vi "Get Least Common Multiple (LCM)-array input.vi"(8 "Error In":errorcluster, 11 "Input integers":i32[](array[numeric])) -> (0 "Error Out":errorcluster, 3 "Least Common Multiple (LCM)":i32)   [LabVIEW 2021, in "Numeric Utilities.lvlib"]
uses:
  Numeric Utilities.lvlib
  Factors cluster.ctl
panel:
  out "Loop iteration":i32
  # "Development\ncontrols/indicators useful for development and testing, but which are not outputs of the VI"
  # "Input\nInputs to the VI"
  # "Output\nOutputs of the VI"
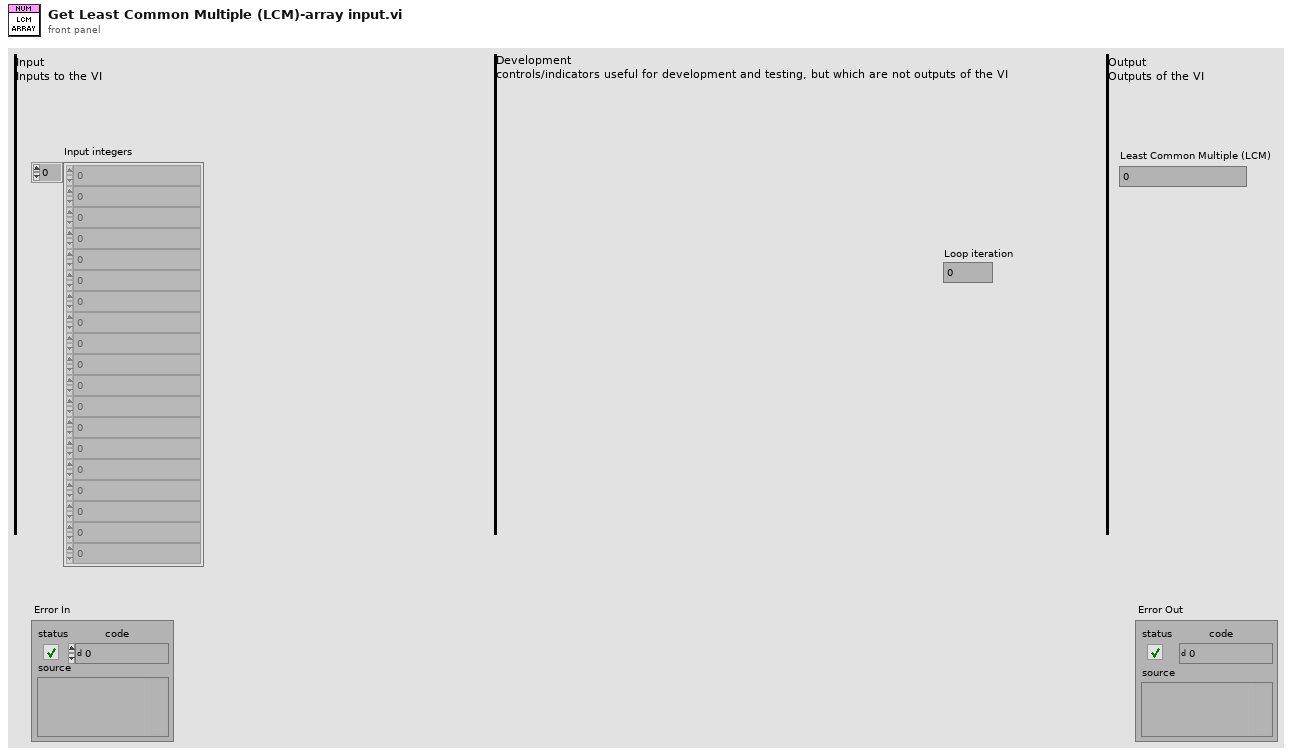
[diagram p1: front panel]
types:
  T1 = typedef "Numeric Utilities.lvlib/Factors cluster.ctl" = cluster{"Factor":i32, "Power":i32}
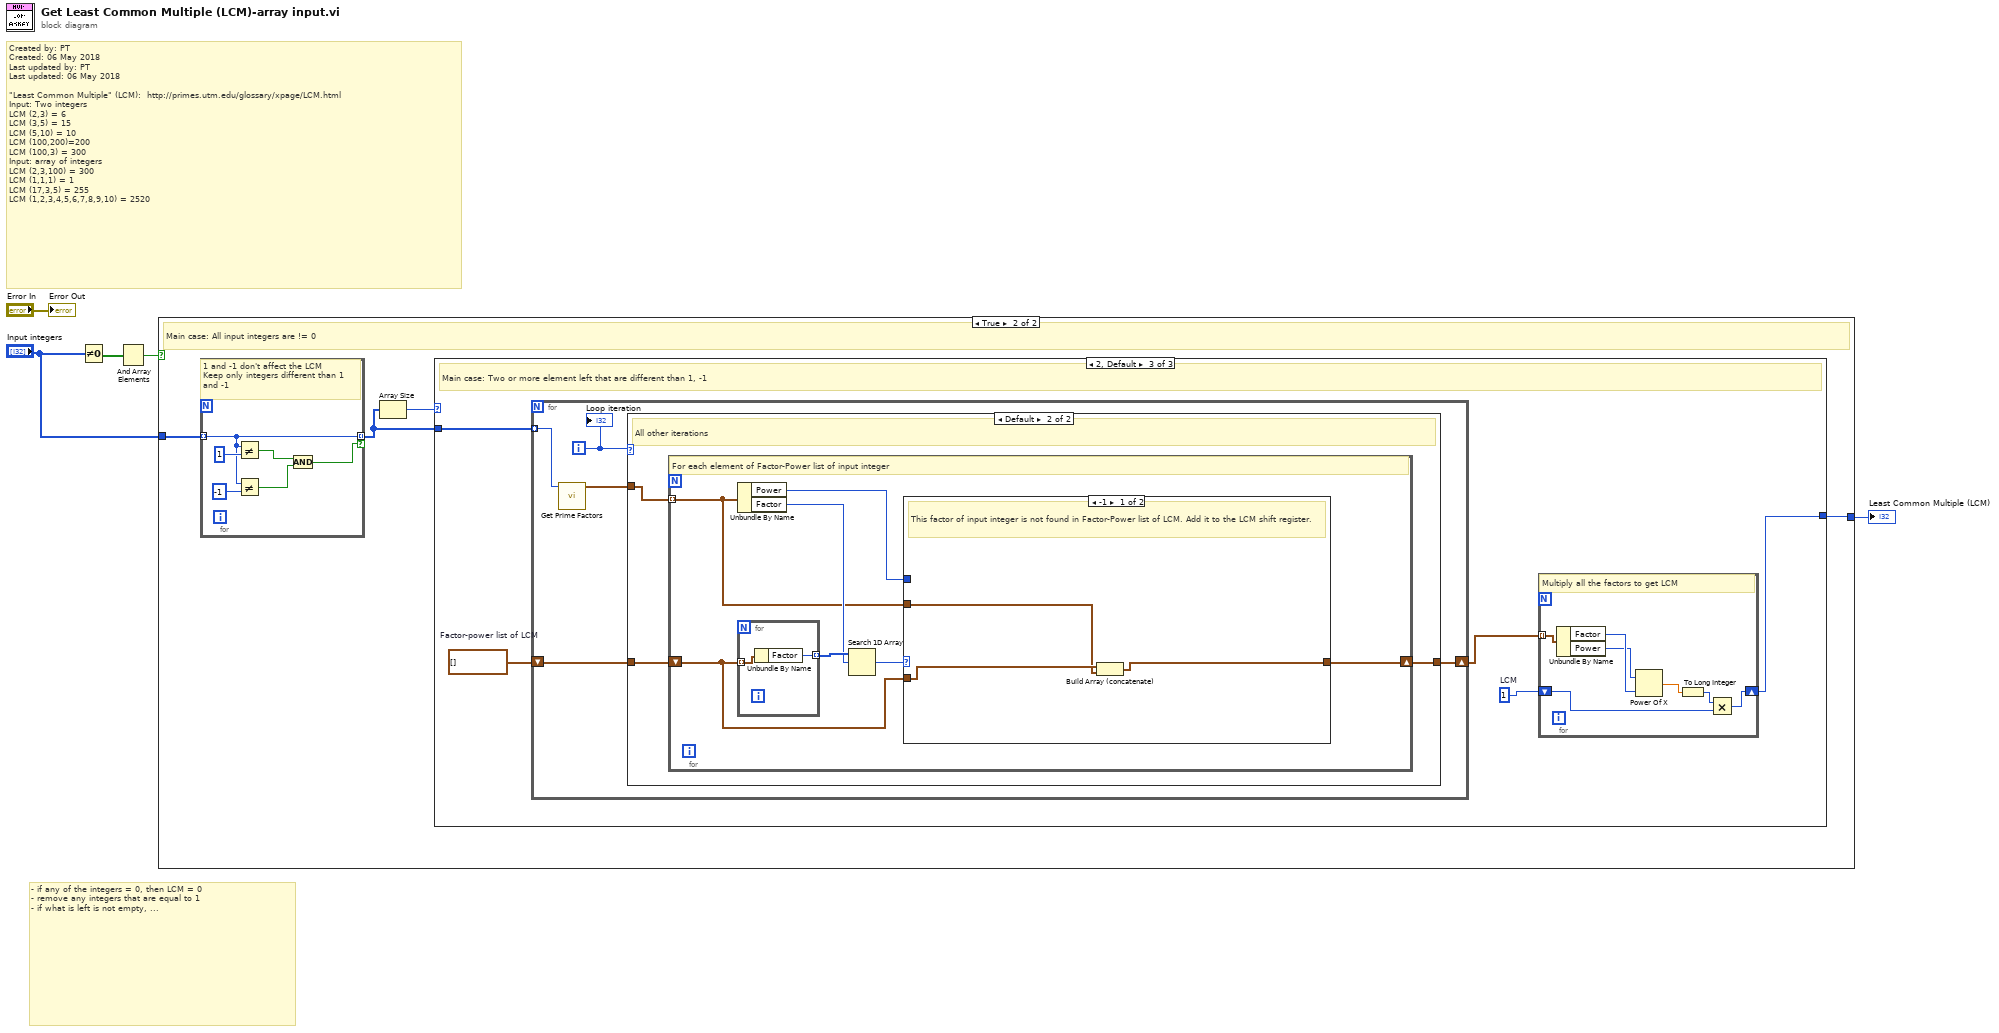
[diagram p0: block diagram]
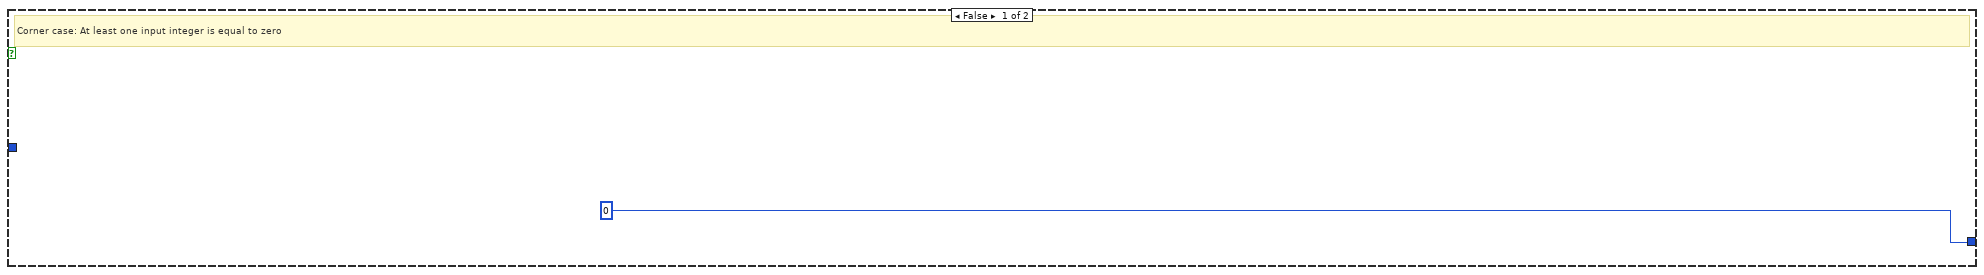
[diagram p2: hidden frame]
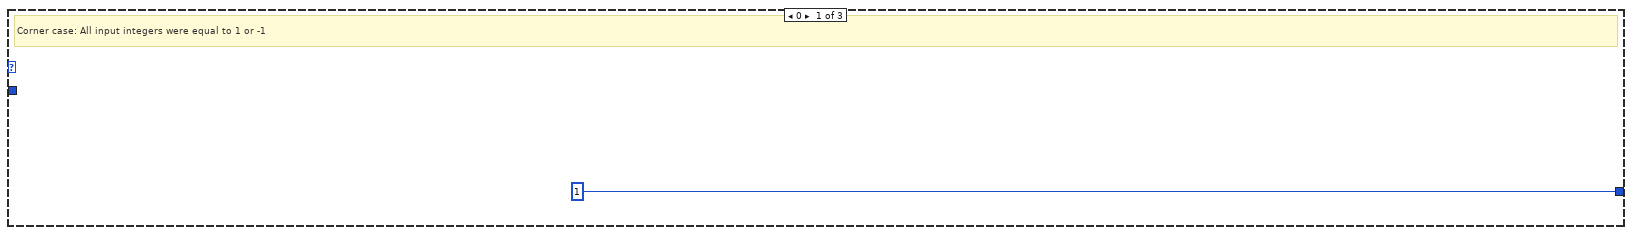
[diagram p3: hidden frame]
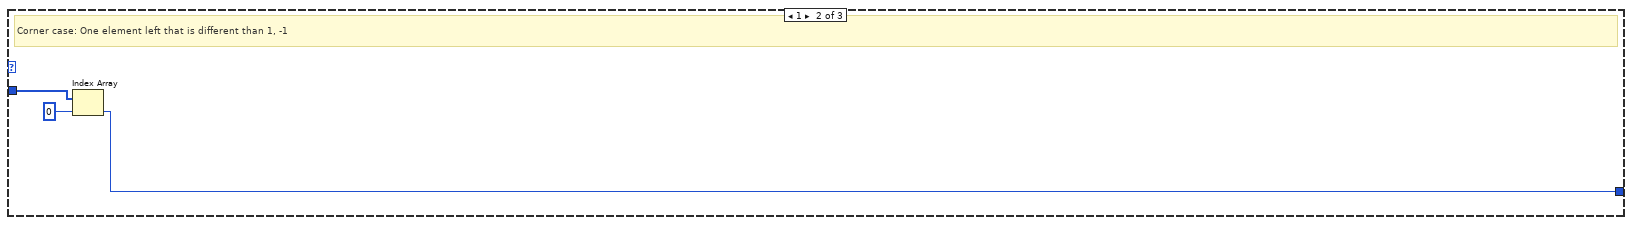
[diagram p4: hidden frame]
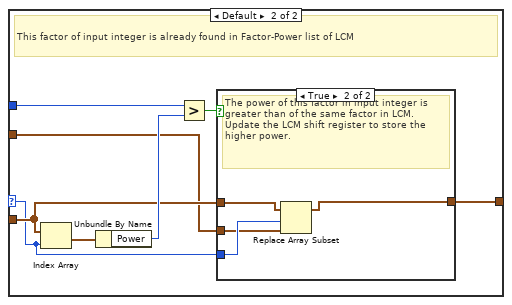
[diagram p6: hidden frame]
diagram:
  # "- if any of the integers = 0, then LCM = 0\n- remove any integers that are equal to 1\n- if what is left is not empty, ..."
  # "Created by: PT\nCreated: 06 May 2018\nLast updated by: PT\nLast updated: 06 May 2018\n\n\"Least Common Multiple\" (LCM):  http://primes.utm.edu/glossary/xpage/LCM.html\nInput: Two integers\nLCM (2,3) = 6\nLCM (3,5) = 15\nLCM (5,10) = 10\nLCM (100,200)=200\nLCM (100,3) = 300\nInput: array of integers\nLCM (2,3,100) = 300\nLCM (1,1,1) = 1\nLCM (17,3,5) = 255 \nLCM (1,2,3,4,5,6,7,8,9,10) = 2520"
  n1 = Not Equal To 0?(x="Input integers") -> (x != 0?=w4:bool[])
  n2 = And Array Elements(Boolean array=w4) -> (logical AND=w3:bool)
  n3 = case shown="True" w3 {
    tunnel: [0 w8] -> w2
    tunnel: "Input integers" -> [_ w10]
    frame False {
      # "Corner case: At least one input integer is equal to zero"
    }
    frame True {
      # "Main case: All input integers are != 0"
      n4 = for {
        tunnel: w10 -> [w63] mode=indexing
        tunnel: [w63] -> w7 mode=indexing if=w65
        # "1 and -1 don't affect the LCM\nKeep only integers different than 1 and -1"
        n5 = Not Equal?(x=w63, y=1) -> (x != y?=w64:bool)
        n6 = Not Equal?(x=w63, y=-1) -> (x != y?=w61:bool)
        n7 = And(x=w64, y=w61) -> (x .and. y?=w65:bool)
      }
      n8 = Array Size(array=w7) -> (size(s)=w9:i32)
      n9 = case shown="2, Default" w9 {
        tunnel: [1 w12 w15] -> w8
        tunnel: w7 -> [_ w14 w19]
        frame 0 {
          # "Corner case: All input integers were equal to 1 or -1"
        }
        frame 1 {
          # "Corner case: One element left that is different than 1, -1"
          n10 = Index Array(array=w14, index=0) -> (element=w12:i32)
        }
        frame 2, Default {
          w17 = 1  # LCM
          w18 = T1[] []  # Factor-power list of LCM
          # "Main case: Two or more element left that are different than 1, -1"
          n11 = for {
            tunnel: w19 -> [w31] mode=indexing
            shift-right: [w28] -> w16
            shift-left: w18 -> [w27]
            i -> [w30]
            n12 = call "Get Prime Factors.vi"("x"=w31) -> ("Factors out"=w29:T1[])  [unwired: 5 in, 5 out]
            n13 = case shown="Default" w30 {
              tunnel: w29 -> [w32 w34]
              tunnel: [w32 w33] -> w28
              tunnel: w27 -> [_ w35]
              frame 0 {
                # "Initialise the Factor-Power list of LCM with the Factor-Power list of the first input integer"
                # "First iteration"
              }
              frame Default {
                # "All other iterations"
                n14 = for {
                  tunnel: w34 -> [w37] mode=indexing
                  shift-right: [w36] -> w33
                  shift-left: w35 -> [w39]
                  # "For each element of Factor-Power list of input integer"
                  n15 = Unbundle By Name(w37) -> ("Power"=w38:i32, "Factor"=w41:i32)
                  n16 = for {
                    tunnel: w39 -> [w60] mode=indexing
                    tunnel: [w59] -> w42 mode=indexing
                    n17 = Unbundle By Name(w60) -> ("Factor"=w59:i32)
                  }
                  n18 = Search 1D Array(1D array=w42, element=w41) -> (index of element=w40:i32)  [unwired: 1 in]
                  n19 = case shown="-1" w40 {
                    selector: w40 -> [_ w48]
                    tunnel: w39 -> [w45 w49]
                    tunnel: w38 -> [_ w51]
                    tunnel: w37 -> [w44 w47]
                    tunnel: [w43 w46] -> w36
                    frame -1 {
                      # "This factor of input integer is not found in Factor-Power list of LCM. Add it to the LCM shift register."
                      n20 = Build Array (concatenate)(w45, w44) -> (w43:T1[])
                    }
                    frame Default {
                      # "This factor of input integer is already found in Factor-Power list of LCM"
                      n21 = Index Array(array=w49, index=w48) -> (element=w52:T1)
                      n22 = Unbundle By Name(w52) -> ("Power"=w50:i32)
                      n23 = Greater?(x=w51, y=w50) -> (0:w53:bool)
                      n24 = case shown="True" w53 {
                        tunnel: w49 -> [w54 w58]
                        tunnel: w48 -> [_ w57]
                        tunnel: w47 -> [_ w56]
                        tunnel: [w54 w55] -> w46
                        frame False {
                          # "No need to update LCM shift register"
                        }
                        frame True {
                          # "The power of this factor in input integer is greater than of the same factor in LCM. Update the LCM shift register to store the higher power."
                          n25 = Replace Array Subset(array=w58, new element=w56, index=w57) -> (w55:T1[])
                        }
                      }
                    }
                  }
                }
              }
            }
            "Loop iteration" <- w30
          }
          n26 = for {
            tunnel: w16 -> [w26] mode=indexing
            shift-right: [w20] -> w15
            shift-left: w17 -> [w21]
            # "Multiply all the factors to get LCM"
            n27 = Unbundle By Name(w26) -> ("Factor"=w25:i32, "Power"=w24:i32)
            n28 = Power Of X(1:w25, 2:w24) -> (0:w23:dbl)
            n29 = To Long Integer(number=w23) -> (32bit integer=w22:i32)
            n30 = Multiply(x=w22, y=w21) -> (x*y=w20:i32)
          }
        }
      }
    }
  }
  "Least Common Multiple (LCM)" <- w2
  "Error Out" <- "Error In"
